vi "Pump Module (Main).vi"(7 "Name of Parent Panel":string="Main.vi", 9 "New Center Coords":T1={"Horizontal"=470, "Vertical"=200}, 10 "Config":variant, 11 "Main UI Message Queue":refnum<queue>) -> ()   [LabVIEW 2018, in "Pump Module.lvlib"]
doc: "This Continuous Measurement sample project is based on the Queued Message Handler template.\n\nThe Event Handling Loop generates messages based on user interface actions.\n\nThe Message Handling Loop processes messages generated by the Event Handling Loop, or by other messages. There are also Acquisition and Logging message handling loop subVIs, and a chart updating loop."
uses:
  Pump Module.lvlib
  support/Message Queue/Message Cluster.ctl
  <vilib>/Utility/miscctls.llb/LVPoint32TypeDef.ctl
  controls/UI Data.ctl
  controls/UI State.ctl
  Pump Module State Cluster.ctl
  Pump Module Config Cluster.ctl
  Pump Module Settings Cluster.ctl
  Ismatec ISM 831C/Controls/Ismatech Settings Cluster.ctl
  Masterflex 7550-30/Controls/Settings Cluster.ctl
  VICI M50 Party Mode/Settings Cluster.ctl
  Measure Instrument/PID 2 Output Enum.ctl
  Tacmina QI/Tacmina QI DAQ Setting.ctl
  KNF Pump/Settings Cluster plus SIMDOS.ctl
  ASIA Pump/Pump Settings.ctl
  FLOM Pump/Settings Cluster.ctl
  SSI PR Class/SSI PR Settings Cluster.ctl
  Measure Instrument/State Enum.ctl
  Pump Module Display.ctl
  Sequencing/Squence Update Cluster.ctl
  support/Message Queue/Enqueue Message (Single).vi
  <vilib>/Utility/error.llb/Error Cluster From Error Code.vi
  <vilib>/ErrorRing/Error Ring.xnode
  support/User Event - Stop/User Event - Stop.lvlib
  support/Support Library.lvlib
  support/Message Queue/Message Queue.lvlib
  Measure Instrument/Pump Module Engine.lvlib
  Masterflex 7550-30/Masterflex 7550-30.lvlib
  Ismatec ISM 831C/Ismatec ISM 831C.lvlib
  Measure Instrument/Feed Module Engine.lvlib
  Tacmina QI/Tacmina QI.lvlib
  KNF Pump/KNF SIMDOS.lvlib
  ASIA Pump.lvlib
  Sequencing/Sequencing Library.lvlib
  VICI M50 Party Mode/VICI M6 M50 Party Mode.lvlib
  Pump Settings Dialog.vi
  FLOM Pump/FLOM Pump.lvlib
  support/Command Log VIs/Command Logging.lvlib
  SSI PR Class/SSI PR Pump.lvlib
panel:
  in  "Settings Button":bool
  out "ml/min":dbl format="%#_5g"
  out "PSIG":dbl format="%#_5g"
  out "Sequence Started":bool
  out "ScanCode":i16
  out "Pump %":dbl format="%#_5g"
  out "Ring":u16(ring)=2
  out "Log File path":path
  out "Status":string
  in  "Exit":bool
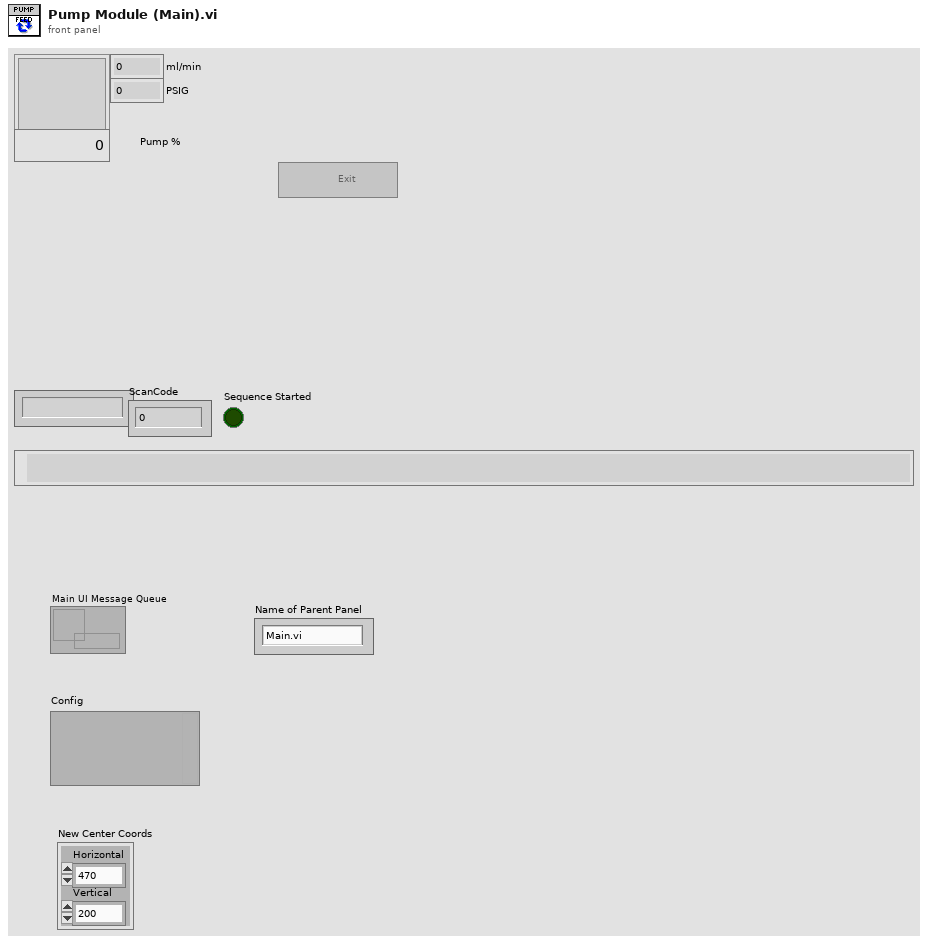
[diagram p1: front panel]
types:
  T1 = typedef "LVPoint32TypeDef.ctl" = cluster{"Horizontal":i32, "Vertical":i32}
  T2 = typedef "Pump Module.lvlib/Pump Module Config Cluster.ctl" = cluster{"GUID":string, "Drop Coords":T1, "Process Name":string, "Queue Name":string, "Settings":T3, "Load Count":i32}
  T3 = typedef "Pump Module.lvlib/Pump Module Settings Cluster.ctl" = cluster{"Cycle Period":dbl, "Ismatech":T4, "Masterflex":T5, "Manual Entry":dbl, "VICI Settings":T6, "Output Device":T7, "Tacmina Settings":T8, "KNF SIMDOS Settings":T9, "ASIA Pump C":T10, "FLOM Settings":T11, "Pump Calibration File":path, "Calibration":dbl, "Pump Cal Enum":u16, "SSI PR Settings":T12}
  T4 = typedef "Ismatec ISM 831C.lvlib/Ismatech Settings Cluster.ctl" = cluster{"VISA resource name":refnum<visa-resource-name>, "Simulated?":bool, "Pump Number":dbl, "Reverse?":bool}
  T5 = typedef "Masterflex 7550-30.lvlib/Settings Cluster.ctl" = cluster{"VISA resource name":refnum<visa-resource-name>, "Simulated?":bool, "Pump Number":dbl, "Reverse?":bool}
  T6 = typedef "VICI M6 M50 Party Mode.lvlib/Settings Cluster.ctl" = cluster{"VISA resource name":refnum<visa-resource-name>, "Simulated?":bool, "Pump Letter":string, "Reverse?":bool}
  T7 = typedef "PID 2 Output Enum.ctl" = enum16{"Default", "Ismatec ISM 831C", "Masterflex 7550-30", "VICI", "Tacmina QI", "KNF SIMDOS", "ASIA Type C", "FLOM UI-22-11", "SSI PR"}
  T8 = typedef "Tacmina QI.lvlib/Tacmina QI DAQ Setting.ctl" = cluster{"Analog DAQ Task":refnum<k21>, "Digital DAQ Task":refnum<k21>}
  T9 = typedef "KNF SIMDOS.lvlib/Settings Cluster plus SIMDOS.ctl" = cluster{"VISA resource name":refnum<visa-resource-name>, "Simulated?":bool}
  T10 = typedef "ASIA Pump.lvlib/Pump Settings.ctl" = cluster{"ASIA Pump #":i32, "channel":i32, "Simulated":bool}
  T11 = typedef "FLOM Pump.lvlib/Settings Cluster.ctl" = cluster{"VISA resource name":refnum<visa-resource-name>, "Simulated?":bool, "Pump Number":dbl}
  T12 = typedef "SSI PR Pump.lvlib/SSI PR Settings Cluster.ctl" = cluster{"VISA resource name":refnum<visa-resource-name>, "Simulated?":bool}
  T13 = typedef "Pump Module.lvlib/Pump Module State Cluster.ctl" = cluster{"Pump Module Config":T2, "State":T14, "Start Time":timestamp, "Current Time":timestamp, "First Iteration":bool, "Data":cluster{"Pump Speed":dbl}, "Process Name":string, "Pump On?":bool}
  T14 = typedef "Feed Module.lvlib/Feed Module Engine.lvlib/State Enum.ctl" = enum16{"Measuring", "Idle", "Paused"}
  T15 = typedef "UI State.ctl" = enum16{"Idle", "Acquiring and Logging", "Waiting for Exit", "Waiting for Exit (Acq Stopped)", "Waiting for Exit (Log Stopped)", "Waiting for Stop", "Waiting for Stop (Acq Stopped)", "Waiting for Stop (Log Stopped)"}
  T16 = typedef "UI Data.ctl" = cluster{"Start Ref":refnum<vi>, "Trigger Ref":refnum<vi>, "Stop Ref":refnum<vi>, "Settings Ref":refnum<vi>, "Status Ref":refnum<vi>, "Exit Ref":refnum<vi>, "Data Ref":refnum<vi>}
  T17 = typedef "Pump Module.lvlib/All Message Queues.ctl" = cluster{"Engine":refnum<queue>, "Pump UI":refnum<queue>, "Pump Engine":refnum<queue>, "Pump Display":refnum<queue>}
  T18 = typedef "Sequencing Library.lvlib/Squence Update Cluster.ctl" = cluster{"Auto?":bool, "Manual Entry":dbl, "Setpoint":dbl}
  T19 = enum8{"Enabled", "Disabled", "Disabled and Grayed Out"}
  T20 = typedef "Pump Module.lvlib/Pump Module Display.ctl" = cluster{"Pump On?":enum16{"Off", "On", "Not Initialized"}, "Cycle Period":dbl, "Current Pump Speed":dbl, "Current Pump Pressure":dbl, "Current Pump Flow":dbl, "Output":T7}
  T21 = cluster{"Shift":bool, "Ctrl":bool, "Alt":bool, "Cmd":bool, "Opt":bool}
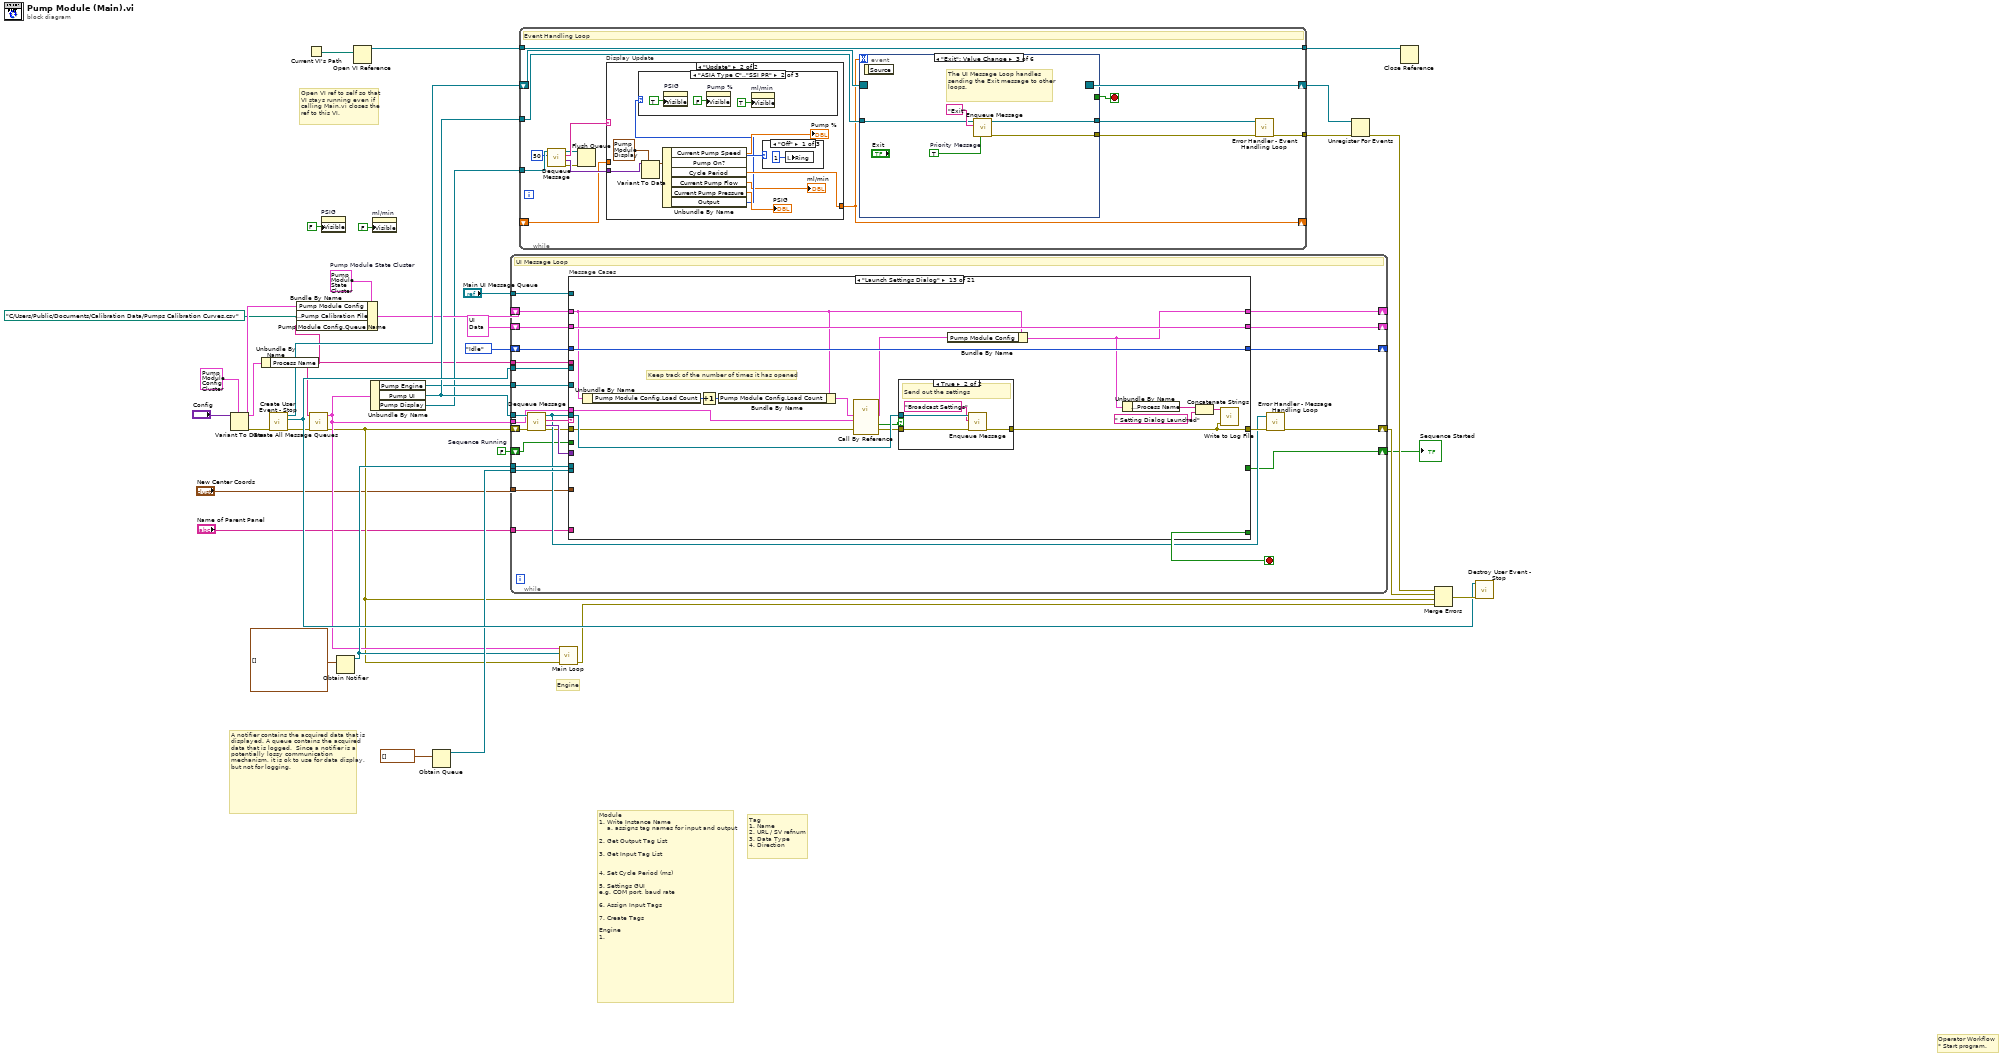
[diagram p0: block diagram]
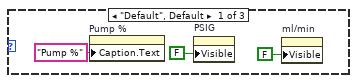
[diagram p3: hidden frame]
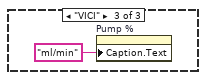
[diagram p4: hidden frame]
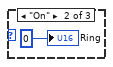
[diagram p5: hidden frame]
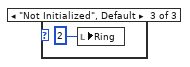
[diagram p6: hidden frame]
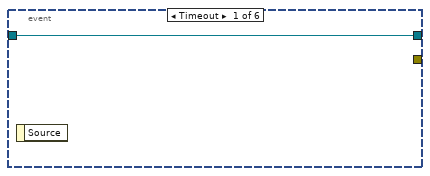
[diagram p7: hidden frame]
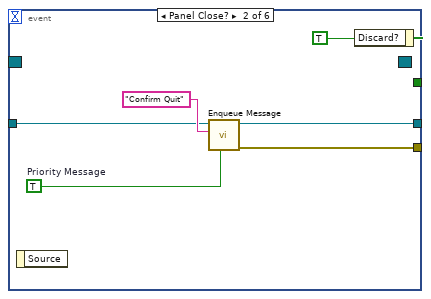
[diagram p8: hidden frame]
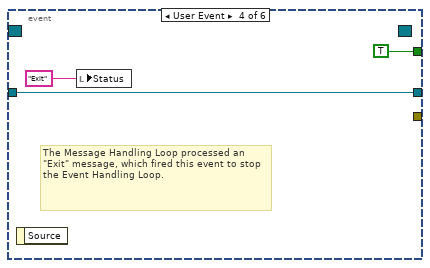
[diagram p9: hidden frame]
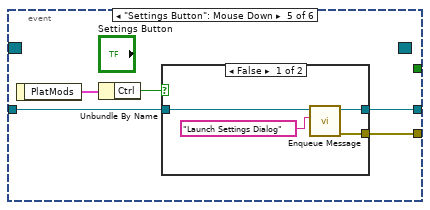
[diagram p10: hidden frame]
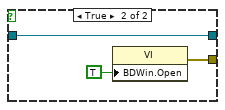
[diagram p11: hidden frame]
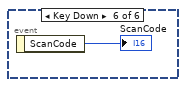
[diagram p12: hidden frame]
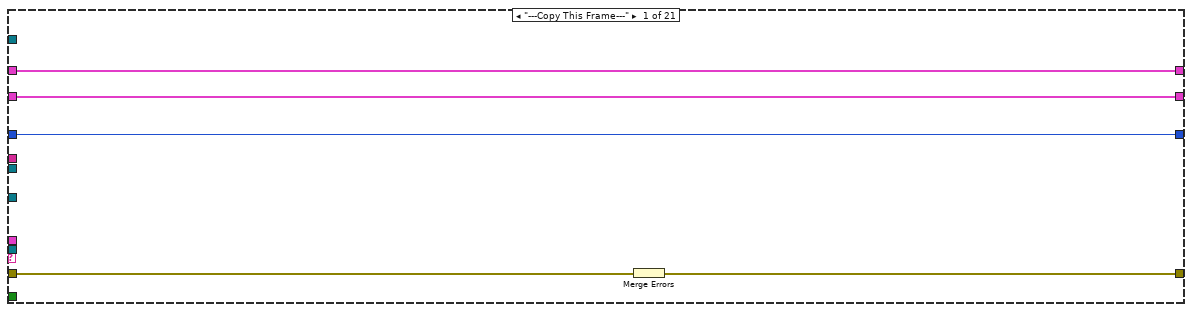
[diagram p13: hidden frame]
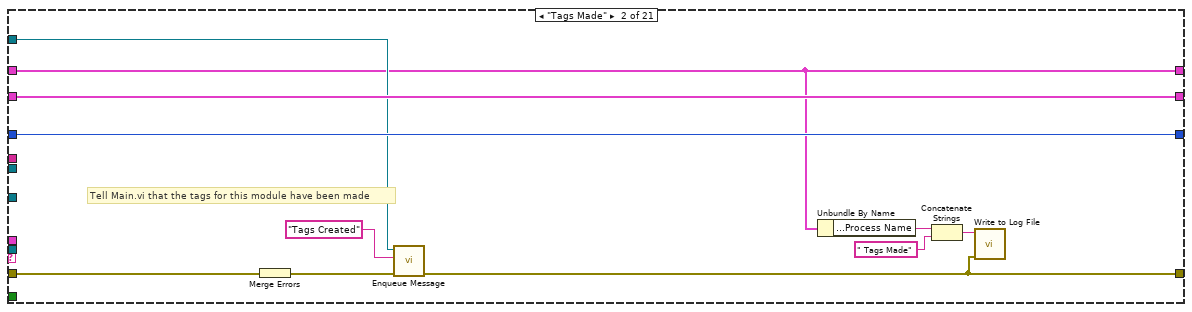
[diagram p14: hidden frame]
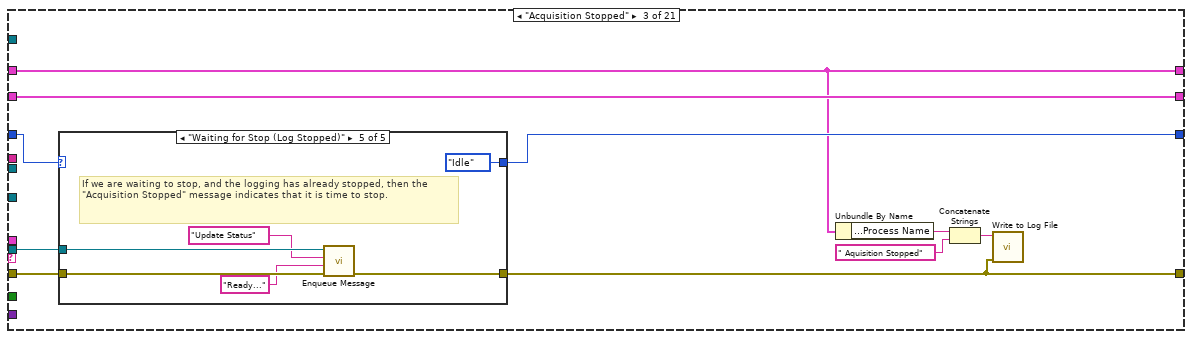
[diagram p15: hidden frame]
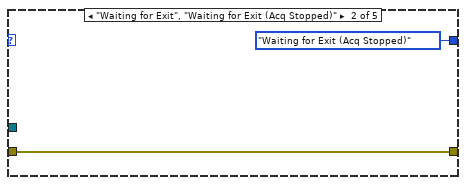
[diagram p17: hidden frame]
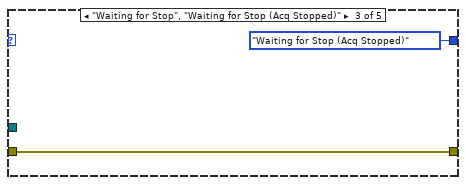
[diagram p18: hidden frame]
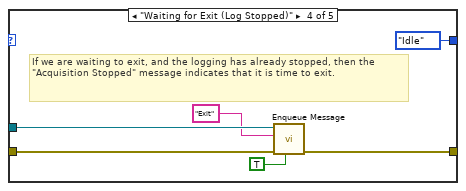
[diagram p19: hidden frame]
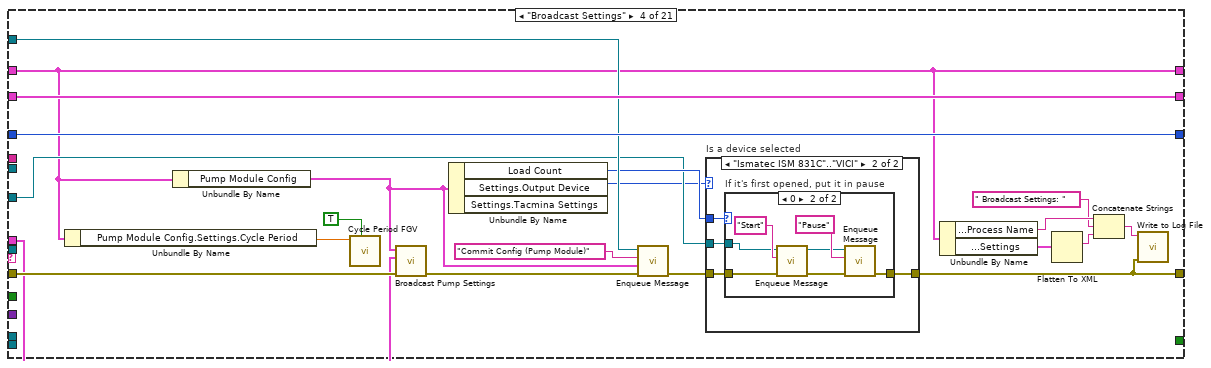
[diagram p20: hidden frame]
diagram:
  w5 = FALSE  # Sequence Running
  w15 = T13 {"Pump Module Config"={"GUID"="", "Drop Coords"={"Horizontal"=0, "Vertical"=0}, "Process Name"="", "Queue Name"="", "Settings"={"Cycle Period"=500.0, "Ismatech"={"VISA resource name"="", "Simulated?"=TRUE, "Pump Number"=1.0, "Reverse?"=FALSE}, "Masterflex"={"VISA resource name"="", "Simulated?"=TRUE, "Pump Number"=1.0, "Reverse?"=FALSE}, "Manual Entry"=0.0, "VICI Settings"={"VISA resource name"="", "Simulated?"=TRUE, "Pump Letter"="", "Reverse?"=FALSE}, "Output Device"=enum."VICI", "Tacmina Settings"={"Analog DAQ Task"="", "Digital DAQ Task"=""}, "KNF SIMDOS Settings"={"VISA resource name"="", "Simulated?"=TRUE}, "ASIA Pump C"={"ASIA Pump #"=0, "channel"=0, "Simulated"=FALSE}, "FLOM Settings"={"VISA resource name"="", "Simulated?"=TRUE, "Pump Number"=0.0}, "Pump Calibration File"=path "", "Calibration"=0.0, "Pump Cal Enum"=0, "SSI PR Settings"={"VISA resource name"="", "Simulated?"=FALSE}}, "Load Count"=0}, "State"=enum."Idle", "Start Time"=timestamp(0 s since 1904-01-01), "Current Time"=timestamp(0 s since 1904-01-01), "First Iteration"=FALSE, "Data"={"Pump Speed"=0.0}, "Process Name"="", "Pump On?"=FALSE}  # Pump Module State Cluster
  # "Open VI ref to self so that\nVI stays running even if\ncalling Main.vi closes the\nref to this VI."
  # "Engine"
  # "Operator Workflow\n* Start program."
  # "Module \n1. Write Instance Name\n    a. assigns tag names for input and output\n\n2. Get Output Tag List\n\n3. Get Input Tag List\n\n\n4. Set Cycle Period (ms)\n\n5. Settings GUI\ne.g. COM port, baud rate\n\n6. Assign Input Tags\n\n7. Create Tags\n\nEngine\n1."
  # "Tag\n1. Name\n2. URL / SV refnum\n3. Data Type\n4. Direction"
  # "A notifier contains the acquired data that is displayed. A queue contains the acquired data that is logged.  Since a notifier is a potentially lossy communication mechanism, it is ok to use for data display, but not for logging."
  n1 = Variant To Data(type=T2 {"GUID"="", "Drop Coords"={"Horizontal"=0, "Vertical"=0}, "Process Name"="", "Queue Name"="", "Settings"={"Cycle Period"=500.0, "Ismatech"={"VISA resource name"="", "Simulated?"=TRUE, "Pump Number"=1.0, "Reverse?"=FALSE}, "Masterflex"={"VISA resource name"="", "Simulated?"=TRUE, "Pump Number"=1.0, "Reverse?"=FALSE}, "Manual Entry"=0.0, "VICI Settings"={"VISA resource name"="", "Simulated?"=TRUE, "Pump Letter"="", "Reverse?"=FALSE}, "Output Device"=enum."VICI", "Tacmina Settings"={"Analog DAQ Task"="", "Digital DAQ Task"=""}, "KNF SIMDOS Settings"={"VISA resource name"="", "Simulated?"=TRUE}, "ASIA Pump C"={"ASIA Pump #"=0, "channel"=0, "Simulated"=FALSE}, "FLOM Settings"={"VISA resource name"="", "Simulated?"=TRUE, "Pump Number"=0.0}, "Pump Calibration File"=path "", "Calibration"=0.0, "Pump Cal Enum"=0, "SSI PR Settings"={"VISA resource name"="", "Simulated?"=FALSE}}, "Load Count"=0} ("Feed Module Config"), Variant="Config") -> (data=w17:T2, error out=w18:errorcluster)  [unwired: 1 in]
  n2 = Unbundle By Name(w17) -> ("Process Name"=w1:string)
  n3 = call "Create User Event - Stop.vi"("error in (no error)"=w18) -> ("error out"=w11:errorcluster, "User Event - Stop"=w34:refnum<user-event>, "Stop Event Registration Refnum"=w35:refnum<event-registration>)  [unwired: 8 in]
  n4 = Bundle By Name(cluster=w15, "Pump Module Config"=w17, "Pump Module Config.Settings.Pump Calibration File"=path "C:/Users/Public/Documents/Calibration Data/Pumps Calibration Curves.csv", "Pump Module Config.Queue Name"=w1) -> (w19:T13)
  n5 = Current VI's Path() -> (path=w20:path)
  n6 = call "Create All Message Queues.vi"("error in (no error)"=w11, "Process Name"=w1) -> ("error out"=w9:errorcluster, "Message Queues"=w10:T17)  [unwired: 8 in]
  n7 = property on="PSIG" class="DigNum (strict)"("Visible"=FALSE) -> ()  [unwired: 2 in, 2 out]
  n8 = Obtain Notifier(notification data type=waveform(dbl)[] []) -> (notifier out=w23:refnum<notifier>)  [unwired: 3 in, 2 out]
  n9 = Open VI Reference(vi path=w20) -> (vi reference=w21:refnum<vi>)  [unwired: 5 in, 1 out]
  n10 = Unbundle By Name(w10) -> ("Pump Engine"=w26:refnum<queue>, "Pump UI"=w30:refnum<queue>, "Pump Display"=w14:refnum<queue>)
  n11 = property on="ml/min" class="DigNum (strict)"("Visible"=FALSE) -> ()  [unwired: 2 in, 2 out]
  n12 = Obtain Queue(element data type=waveform(dbl)[] []) -> (queue out=w25:refnum<queue>)  [unwired: 4 in, 2 out]
  n13 = while {
    tunnel: w30 -> [w59]
    tunnel: w34 -> [w63]
    shift-right: [w53] -> w38
    shift-left: w9 -> [w62]
    shift-right: [w46] -> _
    shift-left: w19 -> [w39]
    shift-right: [w57] -> _
    shift-left: T16 {"Start Ref"=refnum, "Trigger Ref"=refnum, "Stop Ref"=refnum, "Settings Ref"=refnum, "Status Ref"=refnum, "Exit Ref"=refnum, "Data Ref"=refnum} ("Measurement UI Controls") -> [w58]
    tunnel: w23 -> [w56]
    tunnel: w25 -> [w55]
    shift-right: [w50] -> _
    shift-left: UI_State."Idle" ("UI State") -> [w51]
    tunnel: w26 -> [w49]
    tunnel: "Main UI Message Queue" -> [w47]
    tunnel: w10 -> [w45]
    tunnel: w1 -> [w44]
    tunnel: "New Center Coords" -> [w43]
    tunnel: "Name of Parent Panel" -> [w42]
    shift-right: [w41] -> w6
    shift-left: w5 -> [w40]
    stop <- w64 stop-if-true
    # "UI Message Loop"
    n14 = call "Dequeue Message.vi"("error in (no error)"=w62, "Message Queue"=w59) -> ("error out"=w48:errorcluster, "Message Data"=w60:variant, "Message"=w61:string, "dup Message Queue"=w52:refnum<queue>)  [unwired: 6 in]
    n15 = case "Message Cases" shown="\"Launch Settings Dialog\"" w61 {
      selector: w61 -> [_ _ _ _ _ _ _ _ _ _ _ _ _ _ _ _ _ _ _ _ w508]
      tunnel: w52 -> [_ _ w86 _ w151 w166 _ w229 w243 w270 _ w304 w323 w338 w374 w409 _ _ w466 _ _]
      tunnel: w48 -> [w69 w80 w87 w125 w149 w165 w197 w210 w247 w274 w289 w299 w321 w339 w372 w408 w430 w448 w468 w501 _]
      tunnel: [w68 w71 w82 w112 w145 w163 w198 w204 w232 w250 w289 w291 w311 w333 w362 w394 w436 w443 w460 w502 w510] -> w54
      tunnel: [_ _ _ _ _ _ _ _ _ TRUE _ _ _ _ _ _ _ _ _ _ _] -> w64
      tunnel: w60 -> [_ _ _ _ w152 _ w200 _ w246 w258 _ _ _ _ _ _ _ _ _ w500 _]
      tunnel: w63 -> [_ _ _ _ _ _ _ _ _ w273 _ _ _ _ _ _ _ _ _ _ _]
      tunnel: w39 -> [w65 w70 w81 w111 w154 w162 w195 w208 w234 w249 w280 w290 w322 w334 w366 w404 w428 w442 w470 w491 w509]
      tunnel: w58 -> [w67 w79 w90 w129 w153 w168 w202 w226 w248 w271 w288 w300 w327 w342 w369 w405 w435 w453 w486 w497 w515]
      tunnel: [w67 w79 w90 w129 w153 w168 w202 w226 w248 w271 w287 w300 w327 w342 w369 w405 w435 w453 w486 w497 w515] -> w57
      tunnel: w56 -> [_ _ _ _ _ _ _ _ _ w269 _ _ _ _ _ _ _ _ _ _ _]
      tunnel: w55 -> [_ _ _ _ _ _ _ _ _ w265 _ _ _ _ _ _ _ _ _ _ _]
      tunnel: w51 -> [w66 w78 w89 w128 w155 w167 w196 w215 w238 _ _ _ w326 w341 _ _ _ _ w475 w492 w514]
      tunnel: [w66 w78 w88 w128 w155 w164 w196 w216 w238 UI_State."Idle" ("UI State") UI_State."Idle" ("UI State") UI_State."Idle" ("UI State") w326 w340 UI_State."Acquiring and Logging" ("UI State") UI_State."Acquiring and Logging" ("UI State") UI_State."Acquiring and Logging" ("UI State") UI_State."Acquiring and Logging" ("UI State") w476 w492 w514] -> w50
      tunnel: w49 -> [_ _ _ w117 _ _ _ w214 _ w257 _ _ _ _ _ _ w433 w451 w474 _ _]
      tunnel: w47 -> [_ w75 _ w124 _ _ _ _ _ w259 _ _ _ _ _ _ _ _ _ _ _]
      tunnel: [w65 w70 w81 w111 w143 w162 w195 w203 w234 w249 w280 w290 w312 w334 w361 w393 w428 w442 w459 w491 w509] -> w46
      tunnel: w45 -> [_ _ _ w121 _ _ _ _ _ _ _ _ w320 _ _ _ _ _ _ _ _]
      tunnel: w44 -> [_ _ _ _ _ _ _ _ _ _ _ w295 _ _ _ _ _ _ _ _ _]
      tunnel: w43 -> [_ _ _ _ _ _ _ _ _ _ _ w297 _ _ _ _ _ _ _ _ _]
      tunnel: w42 -> [_ _ _ _ _ _ _ _ _ _ _ w296 _ _ _ _ _ _ _ _ _]
      tunnel: [_ _ _ _ _ _ _ _ _ _ _ _ _ _ _ w402 _ _ _ _ _] -> w41
      tunnel: w40 -> [_ _ _ _ _ _ _ _ _ _ _ _ _ _ _ w398 _ _ _ _ _]
      frame "---Copy This Frame---" {
        # "Duplicate this frame when creating new messages.  Change this comment in the duplicated frame to describe this message."
        n16 = Merge Errors(w69) -> (w68:errorcluster)
      }
      frame "Tags Made" {
        # "Tell Main.vi that the tags for this module have been made"
        # "Duplicate this frame when creating new messages.  Change this comment in the duplicated frame to describe this message."
        n17 = Merge Errors(w80) -> (w76:errorcluster)
        n18 = call-poly "Enqueue Message.vi"("error in (no error)"=w76, "Message"="Tags Created", "Message Queue"=w75) -> ("error out"=w71:errorcluster)  [unwired: 7 in, 1 out]
        n19 = Unbundle By Name(w70) -> ("Pump Module Config.Process Name"=w74:string)
        n20 = Concatenate Strings(w74, " Tags Made" ("text")) -> (w72:string)
        n21 = call "Write to Log File.vi"("error in"=w71, "text"=w72) -> ()  [unwired: 9 in, 1 out]
      }
      frame "Acquisition Stopped" {
        # "Logic for determining what action to take when the acquisition has stopped."
        n22 = case shown="\"Waiting for Stop (Log Stopped)\"" w89 {
          selector: w89 -> [w92 _ _ _ _]
          tunnel: [w92 UI_State."Waiting for Exit (Acq Stopped)" ("UI State") UI_State."Waiting for Stop (Acq Stopped)" ("UI State") UI_State."Idle" ("UI State") UI_State."Idle" ("UI State")] -> w88
          tunnel: w87 -> [w91 w93 w95 w101 w107]
          tunnel: [w91 w93 w95 w100 w106] -> w82
          tunnel: w86 -> [_ _ _ w99 w105]
          frame Default {
          }
          frame "Waiting for Exit", "Waiting for Exit (Acq Stopped)" {
          }
          frame "Waiting for Stop", "Waiting for Stop (Acq Stopped)" {
          }
          frame "Waiting for Exit (Log Stopped)" {
            # "If we are waiting to exit, and the logging has already stopped, then the \"Acquisition Stopped\" message indicates that it is time to exit."
            n23 = call-poly "Enqueue Message.vi"("Priority Message? (F)"=TRUE, "error in (no error)"=w101, "Message"="Exit", "Message Queue"=w99) -> ("error out"=w100:errorcluster)  [unwired: 6 in, 1 out]
          }
          frame "Waiting for Stop (Log Stopped)" {
            # "If we are waiting to stop, and the logging has already stopped, then the \"Acquisition Stopped\" message indicates that it is time to stop."
            n24 = call-poly "Enqueue Message.vi"("error in (no error)"=w107, "Message Data"="Ready..." ("Message"), "Message"="Update Status", "Message Queue"=w105) -> ("error out"=w106:errorcluster)  [unwired: 6 in, 1 out]
          }
        }
        n25 = Unbundle By Name(w81) -> ("Pump Module Config.Process Name"=w85:string)
        n26 = Concatenate Strings(w85, " Aquisition Stopped" ("text")) -> (w83:string)
        n27 = call "Write to Log File.vi"("error in"=w82, "text"=w83) -> ()  [unwired: 9 in, 1 out]
      }
      frame "Broadcast Settings" {
        # "Send the 'Update Settings' message to the Logging and Acquisition message loops."
        n28 = Unbundle By Name(w111) -> ("Pump Module Config.Settings.Cycle Period"=w126:dbl)
        n29 = Unbundle By Name(w111) -> ("Pump Module Config"=w120:T2)
        n30 = call "Cycle Period FGV.vi"("Write"=TRUE, "Cycle Period In (ms)"=w126) -> ()  [unwired: 8 in, 2 out]
        n31 = call "Broadcast Pump Settings.vi"("error in (no error)"=w125, "Message Queues"=w121, "Pump Module Config"=w120) -> ("error out"=w123:errorcluster)  [unwired: 8 in]
        n32 = Unbundle By Name(w120) -> ("Load Count"=w119:i32, "Settings.Output Device"=w116:T7)  [unwired: 1 out]
        n33 = call-poly "Enqueue Message.vi"("error in (no error)"=w123, "Message Data"=w120, "Message"="Commit Config (Pump Module)", "Message Queue"=w124) -> ("error out"=w118:errorcluster)  [unwired: 6 in, 1 out]
        n34 = case "Is a device selected" shown="\"Ismatec ISM 831C\"..\"VICI\"" w116 {
          tunnel: w118 -> [w130 w134]
          tunnel: w117 -> [_ w133]
          tunnel: [w130 w132] -> w112
          tunnel: w119 -> [_ w131]
          frame "Default", Default {
          }
          frame "Ismatec ISM 831C".."VICI" {
            n35 = case "If it's first opened, put it in pause" shown="0" w131 {
              tunnel: w134 -> [w135 w139]
              tunnel: w133 -> [_ w138]
              tunnel: [w135 w142] -> w132
              frame Default {
              }
              frame 0 {
                n36 = call-poly "Enqueue Message.vi"("error in (no error)"=w139, "Message"="Start", "Message Queue"=w138) -> ("error out"=w136:errorcluster, "dup Message Queue"=w137:refnum<queue>)  [unwired: 7 in]
                n37 = call-poly "Enqueue Message.vi"("error in (no error)"=w136, "Message"="Pause", "Message Queue"=w137) -> ("error out"=w142:errorcluster)  [unwired: 7 in, 1 out]
              }
            }
          }
        }
        n38 = Unbundle By Name(w111) -> ("Pump Module Config.Process Name"=w115:string, "Pump Module Config.Settings"=w109:T3)
        n39 = Flatten To XML(anything=w109) -> (xml string=w110:string)
        n40 = Concatenate Strings(w115, " Broadcast Settings: " ("text"), w110) -> (w113:string)
        n41 = call "Write to Log File.vi"("error in"=w112, "text"=w113) -> ()  [unwired: 9 in, 1 out]
      }
      frame "Sequence Update" {
        n42 = Unbundle By Name(w154) -> ("Pump Module Config"=w161:T2)
        n43 = Variant To Data(error in=w149, type=T18 {"Auto?"=TRUE, "Manual Entry"=0.0, "Setpoint"=0.0} ("Cluster"), Variant=w152) -> (data=w159:T18, error out=w148:errorcluster)
        n44 = Unbundle By Name(w159) -> ("Manual Entry"=w158:dbl)
        n45 = Bundle By Name(cluster=w161, "Settings.Manual Entry"=w158) -> (w150:T2)
        n46 = Bundle By Name(cluster=w154, "Pump Module Config"=w150) -> (w143:T13)
        n47 = call-poly "Enqueue Message.vi"("error in (no error)"=w148, "Message"="Broadcast Settings", "Message Queue"=w151) -> ("error out"=w157:errorcluster)  [unwired: 7 in, 1 out]
        n48 = Merge Errors(w157) -> (w145:errorcluster)
        n49 = Unbundle By Name(w143) -> ("Pump Module Config.Process Name"=w147:string)
        n50 = Concatenate Strings(w147, "Sequence Update" ("text")) -> (w144:string)
        n51 = call "Write to Log File.vi"("error in"=w145, "text"=w144) -> ()  [unwired: 9 in, 1 out]
      }
      frame "Confirm Quit" {
        # "Confirm Quit - Message that can confirm whether or not the user wants to exit the application."
        n52 = case shown="\"Acquiring and Logging\"" w167 {
          tunnel: w166 -> [w173 w180]
          tunnel: w165 -> [w172 w178]
          tunnel: [w169 w177] -> w163
          tunnel: [UI_State."Idle" ("UI State") w176] -> w164
          tunnel: w162 -> [_ w175]
          frame Default {
            # "If 'Confirm Quit' comes in while the system is idle, there is no need for a confirmation message."
            n53 = call-poly "Enqueue Message.vi"("Priority Message? (F)"=TRUE, "error in (no error)"=w172, "Message"="Exit", "Message Queue"=w173) -> ("error out"=w169:errorcluster)  [unwired: 6 in, 1 out]
          }
          frame "Acquiring and Logging" {
            n54 = Two Button Dialog(message="Are you sure you want to quit while the acquisition is running?" ("Confirm Quit Message"), 1:"No" ("No"), 2:"Yes" ("Yes")) -> (T button?=w179:bool)
            n55 = case shown="True" w179 {
              tunnel: w180 -> [_ w194]
              tunnel: w178 -> [w184 w193]
              tunnel: [w184 w186] -> w177
              tunnel: [UI_State."Acquiring and Logging" ("UI State") UI_State."Waiting for Exit" ("UI State")] -> w176
              tunnel: w175 -> [_ w187]
              frame False {
                # "User did not want to quit."
              }
              frame True {
                n56 = call-poly "Enqueue Message.vi"("error in (no error)"=w193, "Message"="Stop", "Message Queue"=w194) -> ("error out"=w186:errorcluster)  [unwired: 7 in, 1 out]
                n57 = Unbundle By Name(w187) -> ("Pump Module Config.Process Name"=w189:string)
                n58 = Concatenate Strings(w189, " Quit" ("text")) -> (w190:string)
                n59 = call "Write to Log File.vi"("error in"=w186, "text"=w190) -> ()  [unwired: 9 in, 1 out]
              }
            }
          }
        }
      }
      frame "Display Log File Path" {
        n60 = Variant To Data(error in=w197, type=path "", Variant=w200) -> (data=→"Log File path":path, error out=w198:errorcluster)
      }
      frame "E-Stop" {
        # "Pause the pump when there is an E-STOP"
        # "Message Acquisition and Logging loops to stop"
        # "Enable: Start, Exit, Settings\nDisable: Stop"
        # "Stop the pumps."
        n61 = Unbundle By Name(w226) -> ("Trigger Ref"=w217:refnum<vi>, "Stop Ref"=w218:refnum<vi>, "Start Ref"=w221:refnum<vi>, "Exit Ref"=w220:refnum<vi>, "Settings Ref"=w219:refnum<vi>)
        n62 = call-poly "Enqueue Message.vi"("error in (no error)"=w210, "Message Data"="Ready..." ("Ready..."), "Message"="Update Status", "Message Queue"=w229) -> ("error out"=w212:errorcluster)  [unwired: 6 in, 1 out]
        n63 = Build Array(w221, w220, w219) -> (w224:refnum<vi>[])
        n64 = Build Array(w217, w218) -> (w223:refnum<vi>[])
        n65 = call-poly "Enqueue Message.vi"("error in (no error)"=w212, "Message"="Pause", "Message Queue"=w214) -> ("error out"=w211:errorcluster)  [unwired: 7 in, 1 out]
        n66 = call "Set Enable State on Multiple Controls.vi"("Enable?"=FALSE, "Controls"=w223) -> ()  [unwired: 10 in]
        n67 = call "Set Enable State on Multiple Controls.vi"("Enable?"=TRUE, "Controls"=w224) -> ()  [unwired: 10 in]
        n68 = case shown="Default" w215 {
          selector: w215 -> [_ w231]
          tunnel: [UI_State."Waiting for Stop" ("UI State") w231] -> w216
          frame Default {
          }
          frame "Waiting for Exit" {
          }
        }
        n69 = Merge Errors(w211) -> (w204:errorcluster)
        n70 = Bundle By Name(cluster=w208, "State"=State_Enum."Idle") -> (w203:T13)
        n71 = Unbundle By Name(w203) -> ("Pump Module Config.Process Name"=w207:string)
        n72 = Concatenate Strings(w207, " E-STOP" ("text")) -> (w205:string)
        n73 = call "Write to Log File.vi"("error in"=w204, "text"=w205) -> ()  [unwired: 9 in, 1 out]
      }
      frame "Error" {
        # "Error - Check the error message data and respond accordingly. This message is sent by the \"Error Handler\" VIs at the end of each loop in this application."
        n74 = Variant To Data(error in=w247, type=errorcluster {"status"=FALSE, "code"=0, "source"=""} ("error out"), Variant=w246) -> (data=w244:errorcluster, error out=w240:errorcluster)
        n75 = call <vilib>:"General Error Handler.vi"("error in (no error)"=w244) -> ("message"=w233:string)  [unwired: 10 in, 4 out]
        n76 = call-poly "Enqueue Message.vi"("Priority Message? (F)"=TRUE, "Message"="Exit", "Message Queue"=w243) -> ("error out"=w239:errorcluster)  [unwired: 7 in, 1 out]
        n77 = Merge Errors(w239, w240) -> (w232:errorcluster)
        n78 = Unbundle By Name(w234) -> ("Pump Module Config.Process Name"=w237:string)
        n79 = Concatenate Strings(w237, " Error: " ("text"), w233) -> (w235:string)
        n80 = call "Write to Log File.vi"("error in"=w232, "text"=w235) -> ()  [unwired: 9 in, 1 out]
      }
      frame "Exit" {
        w262 = TRUE  # Delete Module?
        # "Don't check the error outs. The acquisition and logging queues may have already been released."
        # "Close references owned by the Main VI."
        # "Stop the VI"
        # "Exit - Fire the User Event to stop the Event Handling Loop.  Also send Exit messages to the Acquisition and Logging loops."
        n81 = Release Queue(queue=w270, error in (no error)=w274) -> (error out=w268:errorcluster)  [unwired: 1 in, 2 out]
        n82 = call "Fire User Event - Stop.vi"("User Event - Stop"=w273) -> ("error out"=w272:errorcluster)  [unwired: 10 in]
        n83 = Release Notifier(notifier=w269, error in (no error)=w268) -> (error out=w267:errorcluster)  [unwired: 1 in, 2 out]
        n84 = Release Queue(queue=w265, error in (no error)=w267) -> (error out=w266:errorcluster)  [unwired: 1 in, 2 out]
        n85 = call-poly "Enqueue Message.vi"("Message"="Stop", "Message Queue"=w257) -> ("dup Message Queue"=w255:refnum<queue>)  [unwired: 8 in, 1 out]
        n86 = Variant To Data(type=w262, Variant=w258) -> (data=w261:bool, error out=w263:errorcluster)  [unwired: 1 in]
        n87 = Select(t=w262, s=w263, f=w261) -> (s? t:f=w260:bool)
        n88 = call-poly "Enqueue Message.vi"("Message"="Exit", "Message Queue"=w255) -> ()  [unwired: 8 in, 2 out]
        n89 = case "Don't enqueue Delete Module if opening campaign because it\nwill already have been deleted and new config loaded and we create\na race condition." shown="True" w260 {
          tunnel: w259 -> [_ w278]
          tunnel: w249 -> [_ w277]
          frame False {
          }
          frame True {
            n90 = Unbundle By Name(w277) -> ("Pump Module Config.GUID"=w276:string)
            n91 = call-poly "Enqueue Message.vi"("Message Data"=w276, "Message"="Delete Module", "Message Queue"=w278) -> ()  [unwired: 7 in, 2 out]
          }
        }
        n92 = Merge Errors(w272, w266) -> (w250:errorcluster)
        n93 = Unbundle By Name(w249) -> ("Pump Module Config.Process Name"=w253:string)
        n94 = Concatenate Strings(w253, " Exit" ("text")) -> (w251:string)
        n95 = call "Write to Log File.vi"("error in"=w250, "text"=w251) -> ()  [unwired: 9 in, 1 out]
      }
      frame "Init UI Refs" {
        # "Enable: Start, Exit, Settings\nDisable: Stop"
        # "Init UI Refs - Store control references for UI controls.  Also enable/disable controls appropriately."
        n96 = property class="VI"("Front Panel.Closeable"=TRUE ("Front Panel Window:Closeable")) -> ()  [unwired: 2 in, 2 out]
        n97 = control-ref of="Status"() -> (w285:refnum<vi>)
        n98 = control-ref of="Exit"() -> (w282:refnum<vi>)
        n99 = Bundle By Name(cluster=w288, "Status Ref"=w285, "Exit Ref"=w282) -> (w287:T16)
        n100 = Build Array(w282) -> (w284:refnum<vi>[])
        n101 = call "Set Enable State on Multiple Controls.vi"("Enable?"=TRUE, "Controls"=w284) -> ()  [unwired: 10 in]
      }
      frame "Initialize" {
        # "Initialize - Get configuration settings, then message the UI to initialize, and broadcast the settings to the other message loops."
        n102 = property class="VI" props=["FP.State"]() -> (reference out=w298:refnum<vi>)  [unwired: 2 in, 2 out]
        n103 = call-poly "Enqueue Message.vi"("error in (no error)"=w299, "Message"="Init UI Refs", "Message Queue"=w304) -> ("error out"=w302:errorcluster, "dup Message Queue"=w303:refnum<queue>)  [unwired: 7 in]
        n104 = call "Make Child and Move.vi"("Process Name"=w295, "Name of Parent Panel"=w296, "New Center Coords"=w297, "VI in"=w298) -> ()  [unwired: 8 in]
        n105 = call-poly "Enqueue Message.vi"("error in (no error)"=w302, "Message"="Broadcast Settings", "Message Queue"=w303) -> ("error out"=w310:errorcluster, "dup Message Queue"=w309:refnum<queue>)  [unwired: 7 in]
        n106 = call-poly "Enqueue Message.vi"("error in (no error)"=w310, "Message Data"="Ready..." ("Ready..."), "Message"="Update Status", "Message Queue"=w309) -> ("error out"=w291:errorcluster)  [unwired: 6 in, 1 out]
        n107 = Unbundle By Name(w290) -> ("Pump Module Config.Process Name"=w294:string)
        n108 = Concatenate Strings(w294, " Initialize" ("text")) -> (w292:string)
        n109 = call "Write to Log File.vi"("error in"=w291, "text"=w292) -> ()  [unwired: 9 in, 1 out]
      }
      frame "Launch Settings Dialog" {
        # "Keep track of the number of times it has opened"
        # "Launch the Settings Dialog when the user clicks the 'Settings' button."
        n110 = Unbundle By Name(w322) -> ("Pump Module Config.Load Count"=w324:i32)
        n111 = Increment(x=w324) -> (x+1=w325:i32)
        n112 = Bundle By Name(cluster=w322, "Pump Module Config.Load Count"=w325) -> (w319:T13)
        n113 = call-by-ref "?"("error in (no error)"=w321, "Message Queues"=w320, "Pump Module State Cluster In"=w319) -> ("error out"=w317:errorcluster, "Cancelled?"=w316:bool, "Pump Module Config Out"=w318:T2)  [unwired: 7 in, 3 out]
        n114 = case shown="True" w316 {
          tunnel: [w328 w332] -> w311
          tunnel: w323 -> [_ w331]
          tunnel: w317 -> [w328 w329]
          frame False {
          }
          frame True {
            # "Send out the settings"
            n115 = call-poly "Enqueue Message.vi"("error in (no error)"=w329, "Message"="Broadcast Settings", "Message Queue"=w331) -> ("error out"=w332:errorcluster)  [unwired: 7 in, 1 out]
          }
        }
        n116 = Bundle By Name(cluster=w322, "Pump Module Config"=w318) -> (w312:T13)
        n117 = Unbundle By Name(w312) -> ("Pump Module Config.Process Name"=w315:string)
        n118 = Concatenate Strings(w315, " Setting Dialog Launched" ("text")) -> (w313:string)
        n119 = call "Write to Log File.vi"("error in"=w311, "text"=w313) -> ()  [unwired: 9 in, 1 out]
      }
      frame "Logging Stopped" {
        # "Logic for determining what action to take when the logging has stopped."
        n120 = case shown="\"Waiting for Exit (Acq Stopped)\"" w341 {
          selector: w341 -> [w344 _ _ _ _]
          tunnel: [w344 UI_State."Waiting for Exit (Log Stopped)" ("UI State") UI_State."Waiting for Stop (Log Stopped)" ("UI State") UI_State."Idle" ("UI State") UI_State."Idle" ("UI State")] -> w340
          tunnel: w339 -> [w343 w345 w347 w353 w359]
          tunnel: [w343 w345 w347 w352 w358] -> w333
          tunnel: w338 -> [_ _ _ w351 w357]
          frame Default {
          }
          frame "Waiting for Exit", "Waiting for Exit (Log Stopped)" {
          }
          frame "Waiting for Stop", "Waiting for Stop (Log Stopped)" {
          }
          frame "Waiting for Exit (Acq Stopped)" {
            # "If we are waiting to exit, and the acquisition has already stopped, then the \"Logging Stopped\" message indicates that it is time to exit."
            n121 = call-poly "Enqueue Message.vi"("Priority Message? (F)"=TRUE, "error in (no error)"=w353, "Message"="Exit", "Message Queue"=w351) -> ("error out"=w352:errorcluster)  [unwired: 6 in, 1 out]
          }
          frame "Waiting for Stop (Acq Stopped)" {
            # "If we are waiting to stop, and the acquisition has already stopped, then the \"Logging Stopped\" message indicates that it is time to stop."
            n122 = call-poly "Enqueue Message.vi"("error in (no error)"=w359, "Message Data"="Ready..." ("Message"), "Message"="Update Status", "Message Queue"=w357) -> ("error out"=w358:errorcluster)  [unwired: 6 in, 1 out]
          }
        }
        n123 = Unbundle By Name(w334) -> ("Pump Module Config.Process Name"=w337:string)
        n124 = Concatenate Strings(w337, " Logging Stopped" ("text")) -> (w335:string)
        n125 = call "Write to Log File.vi"("error in"=w333, "text"=w335) -> ()  [unwired: 9 in, 1 out]
      }
      frame "Start" {
        # "Clear chart"
        # "Message Acquisition and Logging loops to start"
        # "Enable: Stop\nDisable: Start, Exit, Settings"
        # "Start - Enable/Disable buttons appropriately for an acquisition that has started, and update status display."
        n126 = Unbundle By Name(w369) -> ("Trigger Ref"=w379:refnum<vi>, "Stop Ref"=w380:refnum<vi>, "Start Ref"=w383:refnum<vi>, "Exit Ref"=w382:refnum<vi>, "Settings Ref"=w381:refnum<vi>, "Data Ref"=w371:refnum<vi>)
        n127 = property class="WFChart (strict)"(reference=w371, "History Data"=waveform(dbl)[][] []) -> ()  [unwired: 1 in, 2 out]
        n128 = Build Array(w383, w382, w381) -> (w386:refnum<vi>[])
        n129 = Build Array(w379, w380) -> (w385:refnum<vi>[])
        n130 = call-poly "Enqueue Message.vi"("error in (no error)"=w372, "Message"="Broadcast settings", "Message Queue"=w374) -> ("error out"=w375:errorcluster, "dup Message Queue"=w373:refnum<queue>)  [unwired: 7 in]
        n131 = Unbundle By Name(w366) -> ("State"=w367:T14)
        n132 = call "Set Enable State on Multiple Controls.vi"("Enable?"=TRUE, "Controls"=w385) -> ()  [unwired: 10 in]
        n133 = call "Set Enable State on Multiple Controls.vi"("Enable?"=FALSE, "Controls"=w386) -> ()  [unwired: 10 in]
        n134 = case shown="Default" w367 {
          tunnel: [w388 w391] -> w376
          tunnel: w375 -> [w388 w390]
          tunnel: w373 -> [_ w389]
          frame "Measuring" {
          }
          frame Default {
            # "If it is not started yet, start"
            n135 = call-poly "Enqueue Message.vi"("error in (no error)"=w390, "Message"="Start Loops", "Message Queue"=w389) -> ("error out"=w391:errorcluster)  [unwired: 7 in, 1 out]
          }
        }
        n136 = Merge Errors(w376) -> (w362:errorcluster)
        n137 = Bundle By Name(cluster=w366, "State"=State_Enum."Measuring") -> (w361:T13)
        n138 = Unbundle By Name(w361) -> ("Pump Module Config.Process Name"=w365:string)
        n139 = Concatenate Strings(w365, " Start" ("text")) -> (w363:string)
        n140 = call "Write to Log File.vi"("error in"=w362, "text"=w363) -> ()  [unwired: 9 in, 1 out]
      }
      frame "Sequence Start" {
        # "Clear chart"
        # "Message Acquisition and Logging loops to start"
        # "Enable: Stop\nDisable: Start, Exit, Settings"
        # "Start - Enable/Disable buttons appropriately for an acquisition that has started, and update status display."
        n141 = Unbundle By Name(w405) -> ("Trigger Ref"=w412:refnum<vi>, "Stop Ref"=w413:refnum<vi>, "Start Ref"=w416:refnum<vi>, "Exit Ref"=w415:refnum<vi>, "Settings Ref"=w414:refnum<vi>, "Data Ref"=w407:refnum<vi>)
        n142 = property class="WFChart (strict)"(reference=w407, "History Data"=waveform(dbl)[][] []) -> ()  [unwired: 1 in, 2 out]
        n143 = Build Array(w416, w415, w414) -> (w419:refnum<vi>[])
        n144 = Build Array(w412, w413) -> (w418:refnum<vi>[])
        n145 = call-poly "Enqueue Message.vi"("error in (no error)"=w408, "Message"="Broadcast settings", "Message Queue"=w409) -> ("error out"=w401:errorcluster, "dup Message Queue"=w400:refnum<queue>)  [unwired: 7 in]
        n146 = call "Set Enable State on Multiple Controls.vi"("Enable?"=TRUE, "Controls"=w418) -> ()  [unwired: 10 in]
        n147 = call "Set Enable State on Multiple Controls.vi"("Enable?"=FALSE, "Controls"=w419) -> ()  [unwired: 10 in]
        n148 = case shown="False" w398 {
          selector: w398 -> [_ w426]
          tunnel: [TRUE w426] -> w402
          tunnel: w401 -> [w424 w427]
          tunnel: w400 -> [w422 _]
          tunnel: [w421 w427] -> w399
          frame False {
            # "Start the loop if it isn't started yet"
            n149 = call-poly "Enqueue Message.vi"("error in (no error)"=w424, "Message"="Start Loops", "Message Queue"=w422) -> ("error out"=w421:errorcluster)  [unwired: 7 in, 1 out]
          }
          frame True {
          }
        }
        n150 = Merge Errors(w399) -> (w394:errorcluster)
        n151 = Bundle By Name(cluster=w404, "State"=State_Enum."Measuring") -> (w393:T13)
        n152 = Unbundle By Name(w393) -> ("Pump Module Config.Process Name"=w397:string)
        n153 = Concatenate Strings(w397, " Sequence Start" ("text")) -> (w395:string)
        n154 = call "Write to Log File.vi"("error in"=w394, "text"=w395) -> ()  [unwired: 9 in, 1 out]
      }
      frame "Start Loops" {
        # "I don't think we would have multiple loops but i'm leaving it here incase."
        # "Message Acquisition and Logging loops to start"
        # "Start - Enable/Disable buttons appropriately for an acquisition that has started, and update status display."
        n155 = Unbundle By Name(w428) -> ("Pump Module Config.Process Name"=w429:string)
        n156 = Build Array(w433) -> (w431:refnum<queue>[])
        n157 = for {
          tunnel: w430 -> [w440]
          tunnel: [w439] -> w432 mode=indexing
          tunnel: w431 -> [w438] mode=indexing
          tunnel: w429 -> [w437]
          n158 = call-poly "Enqueue Message.vi"("error in (no error)"=w440, "Message Data"=w437, "Message"="Start", "Message Queue"=w438) -> ("error out"=w439:errorcluster)  [unwired: 6 in, 1 out]
        }
        n159 = property class="VI"("Front Panel.Title"=w429) -> ()  [unwired: 2 in, 2 out]
        n160 = Merge Errors(w432) -> (w436:errorcluster)
      }
      frame "Start Log" {
        # "Message Acquisition and Logging loops to start"
        # "Start - Enable/Disable buttons appropriately for an acquisition that has started, and update status display."
        n161 = Unbundle By Name(w442) -> ("Pump Module Config.Process Name"=w447:string)
        n162 = Build Array(w451) -> (w449:refnum<queue>[])
        n163 = for {
          tunnel: w448 -> [w457]
          tunnel: [w456] -> w450 mode=indexing
          tunnel: w449 -> [w455] mode=indexing
          tunnel: w447 -> [w454]
          n164 = call-poly "Enqueue Message.vi"("error in (no error)"=w457, "Message Data"=w454, "Message"="Start Log", "Message Queue"=w455) -> ("error out"=w456:errorcluster)  [unwired: 6 in, 1 out]
        }
        n165 = property class="VI"("Front Panel.Title"=w447) -> ()  [unwired: 2 in, 2 out]
        n166 = Merge Errors(w450) -> (w443:errorcluster)
        n167 = Unbundle By Name(w442) -> ("Pump Module Config.Process Name"=w446:string)
        n168 = Concatenate Strings(w446, " Start Log" ("text")) -> (w444:string)
        n169 = call "Write to Log File.vi"("error in"=w443, "text"=w444) -> ()  [unwired: 9 in, 1 out]
      }
      frame "Stop" {
        # "Pause the pump when we get a stop command"
        # "Enable: Start, Exit, Settings\nDisable: Stop"
        # "Stop - Enable/Disable buttons appropriately for an acquisition that has stopped, and update status display."
        n170 = Unbundle By Name(w486) -> ("Trigger Ref"=w477:refnum<vi>, "Stop Ref"=w478:refnum<vi>, "Start Ref"=w481:refnum<vi>, "Exit Ref"=w480:refnum<vi>, "Settings Ref"=w479:refnum<vi>)
        n171 = call-poly "Enqueue Message.vi"("error in (no error)"=w468, "Message"="Broadcast settings", "Message Queue"=w466) -> ("error out"=w467:errorcluster, "dup Message Queue"=w465:refnum<queue>)  [unwired: 7 in]
        n172 = Build Array(w481, w480, w479) -> (w484:refnum<vi>[])
        n173 = Build Array(w477, w478) -> (w483:refnum<vi>[])
        n174 = call-poly "Enqueue Message.vi"("error in (no error)"=w467, "Message Data"="Ready..." ("Ready..."), "Message"="Update Status", "Message Queue"=w465) -> ("error out"=w473:errorcluster)  [unwired: 6 in, 1 out]
        n175 = call "Set Enable State on Multiple Controls.vi"("Enable?"=FALSE, "Controls"=w483) -> ()  [unwired: 10 in]
        n176 = call "Set Enable State on Multiple Controls.vi"("Enable?"=TRUE, "Controls"=w484) -> ()  [unwired: 10 in]
        n177 = call-poly "Enqueue Message.vi"("error in (no error)"=w473, "Message"="Pause", "Message Queue"=w474) -> ("error out"=w471:errorcluster)  [unwired: 7 in, 1 out]
        n178 = case shown="Default" w475 {
          selector: w475 -> [_ w490]
          tunnel: [UI_State."Waiting for Stop" ("UI State") w490] -> w476
          frame Default {
          }
          frame "Waiting for Exit" {
          }
        }
        n179 = Merge Errors(w471) -> (w460:errorcluster)
        n180 = Bundle By Name(cluster=w470, "State"=State_Enum."Paused") -> (w459:T13)
        n181 = Unbundle By Name(w459) -> ("Pump Module Config.Process Name"=w463:string)
        n182 = Concatenate Strings(w463, " Stop" ("text")) -> (w461:string)
        n183 = call "Write to Log File.vi"("error in"=w460, "text"=w461) -> ()  [unwired: 9 in, 1 out]
      }
      frame "Update Status" {
        # "Update Display - Convert the message data to a string to display in the Status indicator."
        n184 = Variant To Data(error in=w501, type="", Variant=w500) -> (data=w494:string, error out=w498:errorcluster)
        "Status" <- w494
        n185 = Unbundle By Name(w497) -> ("Trigger Ref"=w493:refnum<vi>, "Stop Ref"=w496:refnum<vi>)
        n186 = property class="Bool"(reference=w496) -> ("DisabledEnum"=w495:T19)  [unwired: 1 in, 2 out]
        n187 = case shown="\"Enabled\"" w495 {
          tunnel: w494 -> [w505 _]
          tunnel: w493 -> [w506 _]
          frame "Enabled" {
            # "Disable the Force Trigger only while we are logging."
            n188 = Build Array(w506) -> (w507:refnum<vi>[])
            n189 = Not Equal?(x="Logging" ("Logging"), y=w505) -> (x != y?=w503:bool)
            n190 = call "Set Enable State on Multiple Controls.vi"("Enable?"=w503, "Controls"=w507) -> ()  [unwired: 10 in]
          }
          frame "Disabled", Default {
          }
        }
        n191 = Merge Errors(w498) -> (w502:errorcluster)
      }
      frame Default {
        # "'Default' case only runs if there is a message that isn't defined in any of the other cases.  Output a programming error."
        n192 = xnode "Error Ring"("parameter 0"=w508) -> ("error out"=w510:errorcluster)
        n193 = Unbundle By Name(w509) -> ("Pump Module Config.Process Name"=w513:string)
        n194 = Concatenate Strings(w513, " Incorrect Message Recieved: " ("text"), w508) -> (w511:string)
        n195 = call "Write to Log File.vi"("error in"=w510, "text"=w511) -> ()  [unwired: 9 in, 1 out]
      }
    }
    n196 = call "Error Handler - Message Handling Loop.vi"("error in (no error)"=w54, "Message Queue"=w52) -> ("dup error in"=w53:errorcluster)  [unwired: 8 in, 1 out]
  }
  "Sequence Started" <- w6
  n197 = while {
    tunnel: w30 -> [w532]
    tunnel: [w534] -> w37
    shift-right: [w533] -> w32
    shift-left: w35 -> [w538]
    tunnel: [w531] -> w22
    tunnel: w21 -> [w531]
    tunnel: w14 -> [w530]
    shift-right: [w527] -> _
    shift-left: _ -> [w526]
    stop <- w537 stop-if-true
    # "Event Handling Loop"
    n198 = call "Dequeue Message.vi"("timeout in ms (-1)"=50, "Message Queue"=w530) -> ("error out"=w523:errorcluster, "Message Data"=w528:variant, "Message"=w529:string, "dup Message Queue"=w524:refnum<queue>)  [unwired: 6 in]
    n199 = Flush Queue(queue=w524, error in (no error)=w523) -> ()  [unwired: 3 out]
    n200 = case "Display Update" shown="\"Update\"" w529 {
      tunnel: w528 -> [_ w548]
      tunnel: [w539 w544] -> w527
      tunnel: w526 -> [w539 _]
      frame "False", Default {
      }
      frame "Update" {
        n201 = Variant To Data(type=T20 {"Pump On?"=enum."Off", "Cycle Period"=500.0, "Current Pump Speed"=0.0, "Current Pump Pressure"=0.0, "Current Pump Flow"=0.0, "Output"=enum."Default"} ("FM Display"), Variant=w548) -> (data=w547:T20)  [unwired: 1 in, 1 out]
        n202 = Unbundle By Name(w547) -> ("Current Pump Speed"=→"Pump %":dbl, "Pump On?"=w545:enum16{"Off", "On", "Not Initialized"}, "Cycle Period"=w544:dbl, "Current Pump Flow"=→"ml/min":dbl, "Current Pump Pressure"=→"PSIG":dbl, "Output"=w541:T7)
        n203 = case shown="\"ASIA Type C\"..\"SSI PR\"" w541 {
          frame "Default", Default {
            n204 = property on="Pump %" class="DigNum (strict)"("Caption.Text"="Pump %" ("Label.Text")) -> ()  [unwired: 2 in, 2 out]
            n205 = property on="PSIG" class="DigNum (strict)"("Visible"=FALSE) -> ()  [unwired: 2 in, 2 out]
            n206 = property on="ml/min" class="DigNum (strict)"("Visible"=FALSE) -> ()  [unwired: 2 in, 2 out]
          }
          frame "ASIA Type C".."SSI PR" {
            n207 = property on="PSIG" class="DigNum (strict)"("Visible"=TRUE) -> ()  [unwired: 2 in, 2 out]
            n208 = property on="Pump %" class="DigNum (strict)"("Visible"=FALSE) -> ()  [unwired: 2 in, 2 out]
            n209 = property on="ml/min" class="DigNum (strict)"("Visible"=TRUE) -> ()  [unwired: 2 in, 2 out]
          }
          frame "VICI" {
            n210 = property on="Pump %" class="DigNum (strict)"("Caption.Text"="ml/min" ("Label.Text")) -> ()  [unwired: 2 in, 2 out]
          }
        }
        n211 = case shown="\"Off\"" w545 {
          frame "Off" {
            n212 = local write "Ring"(u16 1 ("Ring")) -> ()
          }
          frame "On" {
            "Ring" <- u16 0 ("Ring")
          }
          frame "Not Initialized", Default {
            n213 = local write "Ring"(u16 2 ("Ring")) -> ()
          }
        }
      }
    }
    n214 = event shown="[2] \"Exit\": Value Change" {
      selector: w538 -> [_ _ _ _ _ _]
      dyn-events: [_ _ _ _ _ _] -> w533
      timeout: w527 -> [_ _ _ _ _ _]
      tunnel: [_ _ _ TRUE ("Discard?") _ _] -> w537
      tunnel: w532 -> [w559 w562 w567 w571 w576 _]
      tunnel: [_ w560 w570 _ w578 _] -> w535
      tunnel: [w559 w561 w566 w571 w577 _] -> w536
      event Timeout {
        n215 = event-data() -> ()  [unwired: 1 in, 1 out]
      }
      event Panel Close? {
        w563 = TRUE  # Priority Message
        n216 = event-data() -> ()  [unwired: 1 in, 1 out]
        n217 = call-poly "Enqueue Message.vi"("Priority Message? (F)"=w563, "Message"="Confirm Quit", "Message Queue"=w562) -> ("error out"=w560:errorcluster, "dup Message Queue"=w561:refnum<queue>)  [unwired: 7 in]
        n218 = event-data("Discard?"=TRUE) -> ()  [unwired: 1 in, 1 out]
      }
      event "Exit": Value Change {
        w568 = TRUE  # Priority Message
        # "The UI Message Loop handles sending the Exit message to other loops."
        n219 = event-data() -> ()  [unwired: 1 in, 1 out]
        n220 = call-poly "Enqueue Message.vi"("Priority Message? (F)"=w568, "Message"="Exit", "Message Queue"=w567) -> ("error out"=w570:errorcluster, "dup Message Queue"=w566:refnum<queue>)  [unwired: 7 in]
      }
      event User Event {
        # "The Message Handling Loop processed an \"Exit\" message, which fired this event to stop the Event Handling Loop."
        n221 = event-data() -> ()  [unwired: 1 in, 1 out]
        n222 = local write "Status"("Exit" ("Exit String")) -> ()
      }
      event "Settings Button": Mouse Down {
        n223 = event-data() -> ("PlatMods"=w575:T21)  [unwired: 1 in]
        n224 = Unbundle By Name(w575) -> ("Ctrl"=w574:bool)
        n225 = case shown="False" w574 {
          tunnel: [w582 w583] -> w578
          tunnel: [w581 w584] -> w577
          tunnel: w576 -> [w580 w584]
          frame False {
            n226 = call-poly "Enqueue Message.vi"("Message"="Launch Settings Dialog", "Message Queue"=w580) -> ("error out"=w582:errorcluster, "dup Message Queue"=w581:refnum<queue>)  [unwired: 8 in]
          }
          frame True {
            n227 = property class="VI"("BDWin.Open"=TRUE ("Block Diagram Window:Open")) -> (error out=w583:errorcluster)  [unwired: 2 in, 1 out]
          }
        }
      }
      event Key Down {
        n228 = event-data() -> ("ScanCode"=→"ScanCode":i16)  [unwired: 1 in]
      }
    }
    n229 = call "Error Handler - Event Handling Loop.vi"("error in (no error)"=w535, "Message Queue"=w536) -> ("dup error in"=w534:errorcluster)  [unwired: 8 in, 1 out]
  }
  n230 = call "Main Loop.vi"("error in (no error)"=w9, "Chart Notifier"=w23, "Message Queues"=w10) -> ("error out"=w24:errorcluster)  [unwired: 8 in]
  n231 = Unregister For Events(event registration refnum=w32, error in=w37) -> (error out=w33:errorcluster)
  n232 = Close Reference(reference=w22) -> ()  [unwired: 1 in, 1 out]
  n233 = Merge Errors(w33, w38, w9, w24) -> (w36:errorcluster)
  n234 = call "Destroy User Event - Stop.vi"("error in (no error)"=w36, "User Event - Stop"=w34) -> ()  [unwired: 9 in, 1 out]
